vi "hmi.vi"() -> ()   [LabVIEW 2017]
doc: "Demonstrates how to write and receive CAN frames via the Network Interface on the same port. \n\nTo write and receive frames via the Network Interface:\n- select the CAN Network Interface (i.e. CAN0, CAN1, etc.)\n- select the Baud Rate\n- run the VI\n- press the write button to write frames to the can bus\n\nEnable RTR Button to send a Remote Transmission Request or to simply send an empty Frame to request an Answer Frame from a connected device.\n\nEnable Extended Button to write extended Identifier Format. This is done by setting the 30th bit to enable extended format with the driver."
uses:
  <vilib>/nican/nican.llb/ncNetAttr.ctl
panel:
  in  "Tab Control":enum32{"Program", "Settings"}(tab)
  out "ID":u16 format="%04x"
  in  "Device":enum16{"Device 1", "Device 2"}(ring)
  out "Heartbeat":u16 format="%04x"
  in  "shutdown":bool
  in  "IND1":bool
  in  "IND2":bool
  in  "interface":string(combo)="CAN0" caption="Interface"
  # "PRESS AND HOLD"
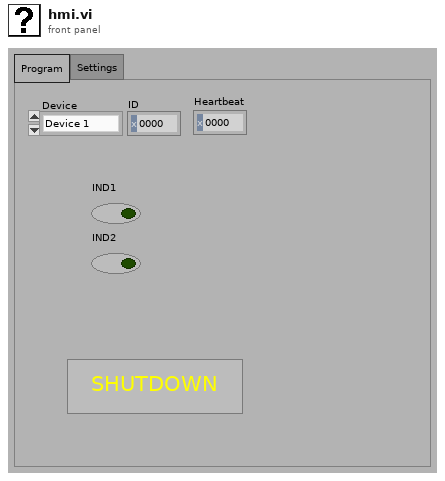
[diagram p1: front panel]
types:
  T1 = typedef "ncNetAttr.ctl" = cluster{"Start On Open":enum32{"FALSE", "TRUE"}, "Baud Rate":u32, "Read Queue Length":u32, "Write Queue Length":u32, "Standard Comparator":u32, "Standard Mask":u32, "Extended Comparator":u32, "Extended Mask":u32}
  T2 = typedef "xobjhandle.ctl" = u32
  T3 = typedef "CanFrameTimed.ctl" = cluster{"Timestamp":dbl, "ArbitrationId":u32, "IsRemote":u8, "DataLength":u8, "Data":u8[]}
  T4 = cluster{dbl, u32, "IsRemote":u8, "DataLength":u8, u8[]}
  T5 = cluster{dbl, u32, "IsRemote":u8, "DataLength":u8, u8[]}[]
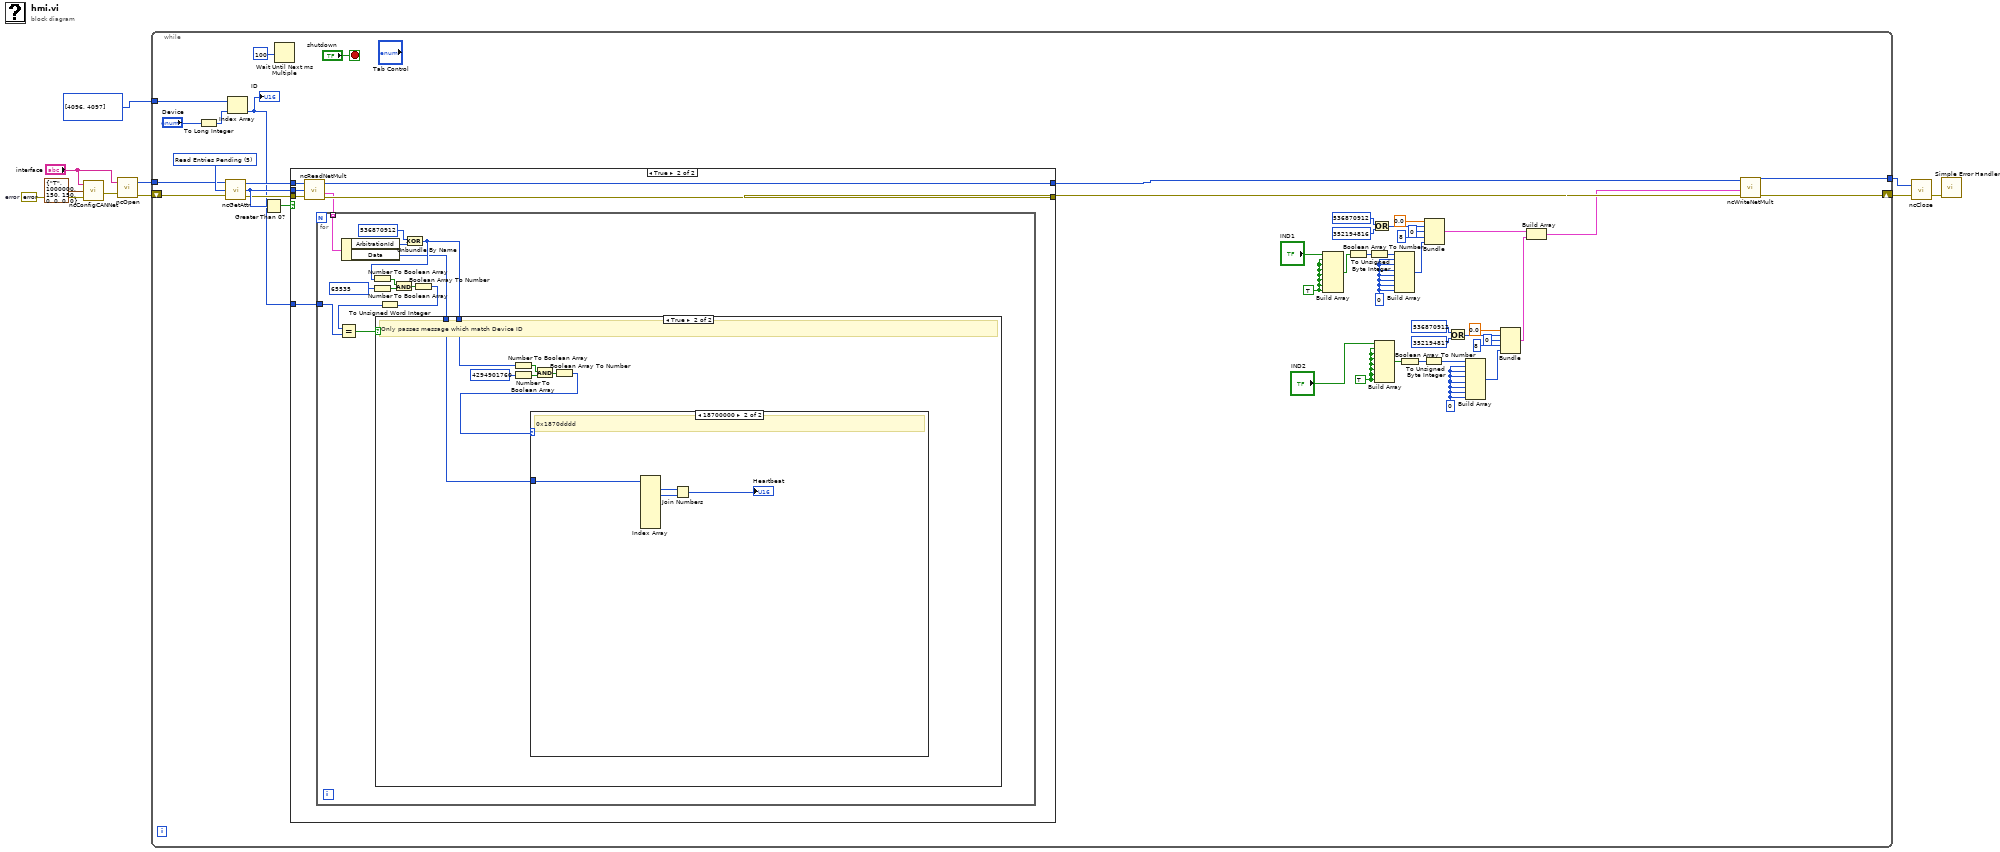
[diagram p0: block diagram]
diagram:
  w6 = errorcluster {"status"=FALSE, "code"=0, "source"=""}  # error
  n1 = call <vilib>:"ncConfigCANNet.vi"("Error in"=w6, "CAN Network Interface Config"=T1 {"Start On Open"=enum."TRUE", "Baud Rate"=1000000, "Read Queue Length"=150, "Write Queue Length"=150, "Standard Comparator"=0, "Standard Mask"=0, "Extended Comparator"=0, "Extended Mask"=0}, "ObjName"="interface") -> ("Error out"=w7:errorcluster)  [unwired: 2 in]
  n2 = call <vilib>:"ncOpen.vi"("Error in"=w7, "ObjName"="interface") -> ("Error out"=w10:errorcluster, "ObjHandle out"=w8:T2)
  n3 = while {
    tunnel: w8 -> [w45]
    tunnel: [w55] -> w3
    shift-right: [w56] -> w2
    shift-left: w10 -> [w44]
    tunnel: u16[] [4096, 4097] -> [w43]
    stop <- "shutdown" stop-if-true
    w19 = TRUE ("element")
    w21 = TRUE ("element")
    w24 = u8 0
    w32 = u8 0
    w48 = u32 5 items=["(reserved)", "Protocol Version", "Software Version", "Object State", "(reserved)", "Read Entries Pending", "Write Entries Pending", "ReadMult Size for Notification", "Listen Only?", "Self Reception?", "Transmit Error Counter", "Receive Error Counter", "Single Shot Transmit?", "Series 2 Filter Mode", "Series 2 Mask", "Series 2 Comparator", "Serial Number", "Form Factor", "Series", "Transceiver Type", "Interface Number", "Series 2 Error/Arb Capture", "Transceiver Mode", "Transceiver External Outputs", "Transceiver External Inputs", "Start Trigger Behavior", "Log Comm Warnings", "User RTSI Frame", "Transmit Mode", "Log Start Trigger?", "Timestamp Format", "Master Timebase Rate", "Virtual Bus Timing"] ("AttrId")
    n4 = To Long Integer(number="Device") -> (32bit integer=w41:i32)
    n5 = call <vilib>:"ncGetAttr.vi"("Error in"=w44, "AttrId"=w48, "ObjHandle in"=w45) -> ("Error out"=w49:errorcluster, "AttrValue"=w52:u32, "ObjHandle out"=w50:T2)
    n6 = Index Array(array=w43, index=w41) -> (element=w40:u16)
    "ID" <- w40
    n7 = Greater Than 0?(x=w52) -> (x > 0?=w51:bool)
    n8 = Wait Until Next ms Multiple(millisecond multiple=u32 100) -> ()  [unwired: 1 out]
    n9 = case shown="True" w51 {
      tunnel: [w57 w65] -> w46
      tunnel: [w58 w64] -> w47
      tunnel: w52 -> [_ w63]
      tunnel: w49 -> [w57 w62]
      tunnel: w50 -> [w58 w61]
      tunnel: w40 -> [_ w59]
      frame False {
      }
      frame True {
        n10 = call <vilib>:"ncReadNetMult.vi"("ObjHandle in"=w61, "Requested Number of Frames"=w63, "Error in"=w62) -> ("ObjHandle out"=w64:T2, "Data"=w60:T3[], "Error out"=w65:errorcluster)  [unwired: 1 out]
        n11 = for {
          tunnel: w60 -> [w78] mode=indexing
          tunnel: w59 -> [w71]
          n12 = Unbundle By Name(w78) -> ("ArbitrationId"=w76:u32, "Data"=w67:u8[])
          n13 = Number To Boolean Array(number=u32 65535 ("y")) -> (Boolean array=w73:bool[])
          n14 = Exclusive Or(1:w76, 2:u32 536870912 ("y")) -> (0:w68:u32)
          n15 = Number To Boolean Array(number=w68) -> (Boolean array=w74:bool[])
          n16 = And(x=w74, y=w73) -> (x .and. y?=w72:bool[])
          n17 = Boolean Array To Number(Boolean array=w72) -> (number=w70:u32)
          n18 = To Unsigned Word Integer(number=w70) -> (unsigned 16bit integer=w66:u16)
          n19 = Equal?(x=w66, y=w71) -> (x = y?=w69:bool)
          n20 = case shown="True" w69 {
            tunnel: w68 -> [_ w80]
            tunnel: w67 -> [_ w85]
            frame False {
            }
            frame True {
              # "Only passes message which match Device ID"
              n21 = Number To Boolean Array(number=w80) -> (Boolean array=w82:bool[])
              n22 = Number To Boolean Array(number=u32 4294901760 ("y")) -> (Boolean array=w83:bool[])
              n23 = And(x=w82, y=w83) -> (x .and. y?=w84:bool[])
              n24 = Boolean Array To Number(Boolean array=w84) -> (number=w79:u32)
              n25 = case shown="18700000" w79 {
                tunnel: w85 -> [_ w86]
                frame Default {
                }
                frame 409993216 {
                  # "0x1870dddd"
                  n26 = Index Array(array=w86) -> (element #1=w88:u8, element #2=w89:u8)  [unwired: 8 in, 6 out]
                  n27 = Join Numbers(hi=w88, lo=w89) -> ((hi.lo)=→"Heartbeat":u16)
                }
              }
            }
          }
        }
      }
    }
    n28 = Build Array("IND1", w21, w21, w21, w21, w21, w21, w21) -> (w15:bool[])
    n29 = Boolean Array To Number(Boolean array=w15) -> (number=w17:u32)
    n30 = To Unsigned Byte Integer(number=w17) -> (unsigned 8bit integer=w16:u8)
    n31 = Or(x=u32 536870912 ("y"), y=u32 352194816) -> (x .or. y?=w30:u32)
    n32 = Build Array("IND2", w19, w19, w19, w19, w19, w19, w19) -> (w20:bool[])
    n33 = Build Array(w16, w24, w24, w24, w24, w24, w24, w24) -> (w26:u8[])
    n34 = Boolean Array To Number(Boolean array=w20) -> (number=w13:u32)
    n35 = To Unsigned Byte Integer(number=w13) -> (unsigned 8bit integer=w14:u8)
    n36 = Bundle(0.0, w30, "IsRemote"=u8 0, "DataLength"=u8 8, w26) -> (w23:T4)  [unwired: 1 in]
    n37 = Or(x=u32 536870912 ("y"), y=u32 352194817) -> (x .or. y?=w38:u32)
    n38 = Build Array(w14, w32, w32, w32, w32, w32, w32, w32) -> (w34:u8[])
    n39 = Bundle(0.0, w38, "IsRemote"=u8 0, "DataLength"=u8 8, w34) -> (w12:T4)  [unwired: 1 in]
    n40 = Build Array(w23, w12) -> (w11:T5)
    n41 = call <vilib>:"ncWriteNetMult.vi"("Error in"=w46, "Data"=w11, "ObjHandle in"=w47) -> ("Error out"=w56:errorcluster, "ObjHandle out"=w55:T2)  [unwired: 7 in]
  }
  n42 = call <vilib>:"ncClose.vi"("Error in"=w2, "ObjHandle in"=w3) -> ("Error out"=w4:errorcluster)  [unwired: 1 in]
  n43 = call <vilib>:"Simple Error Handler.vi"("error in (no error)"=w4) -> ()  [unwired: 4 in, 5 out]
